vi "Get SQL formatted value.vi"(8 "error in (no error)":errorcluster, 11 "Timestamp Column in":refnum<class "Timestamp Column.lvclass">) -> (0 "error out":errorcluster, 2 "Formatted Value":string, 3 "Timestamp Column out":refnum<class "Timestamp Column.lvclass">)   [LabVIEW 2020, in "Basic Columns.lvlib" / "Timestamp Column.lvclass"]
uses:
  Timestamp Column.lvclass
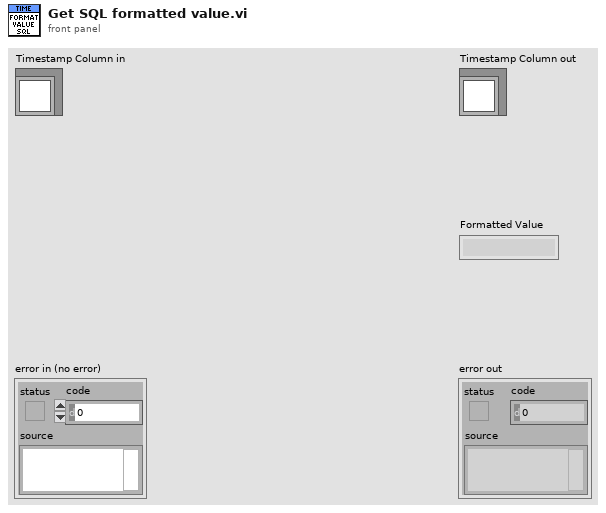
[diagram p1: front panel]
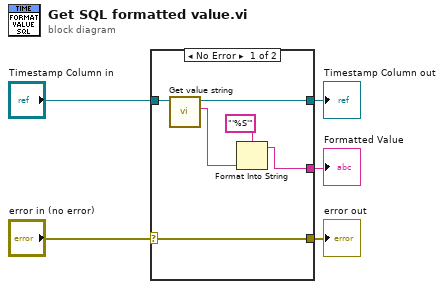
[diagram p0: block diagram]
diagram:
  n1 = case shown="No Error" "error in (no error)" {
    selector: "error in (no error)" -> [w8 w13]
    tunnel: [w8 w13] -> w3
    tunnel: [w11 w12] -> w1
    tunnel: [w9 _] -> w2
    tunnel: "Timestamp Column in" -> [w7 w12]
    frame No Error {
      n2 = call-dynamic "Get value string.vi"("Column in"=w7) -> ("Value"=w6:string, "Column out"=w11:refnum<class "Timestamp Column.lvclass">)  [unwired: 8 in, 1 out]
      n3 = Format Into String(format string="'%S'", w6) -> (resulting string=w9:string)  [unwired: 2 in, 1 out]
    }
    frame Error {
    }
  }
  "error out" <- w3
  "Timestamp Column out" <- w1
  "Formatted Value" <- w2
